vi "Reference_new version_1.0.vi"(1 "Phase log in":dbl=0.9999999999996251, 2 "AI Block Size":i32=40000, 4 "Phase&time":T1, 5 "Reset":bool, 6 "Frequency":dbl=20.0 format="%.2f", 7 "Ref Shape":enum16{"Sine", "Square"}(ring), 8 "Ref Amp":dbl=5.0 format="%.2f", 9 "AI Rate":dbl=200000.0) -> (0 "Ref out":T2={"Ref X"=array[40000 elements], "Ref Y"=array[40000 elements], "AI Rate"=200000.0, "AI Block Size"=40000.0, "Frequency"=20.0, "Ref amp"=5.0} {"Ref amp" step=0.001 format="%0.4f"; "Frequency" step=0.001 format="%0.4f"; "AI Block Size" step=0.001 format="%0.4f"; "AI Rate" step=0.001 format="%0.4f"}, 3 "Phase log":dbl=0.9999999999996251)   [LabVIEW 2013]
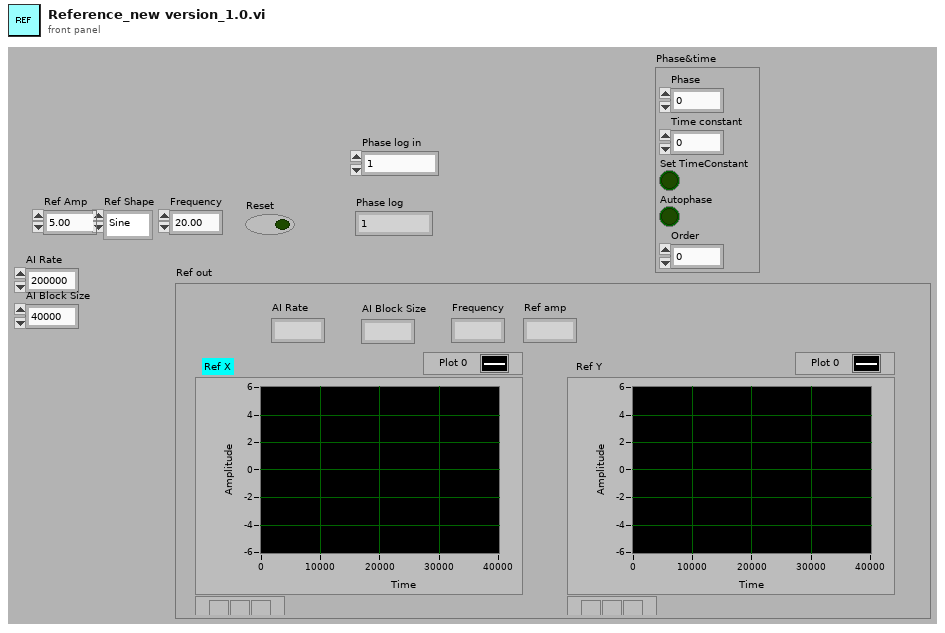
[diagram p1: front panel]
types:
  T1 = cluster{"Phase":dbl, "Time constant":dbl, "Set TimeConstant":bool, "Autophase":bool, "Order":dbl}
  T2 = cluster{"Ref X":dbl[], "Ref Y":dbl[], "AI Rate":dbl, "AI Block Size":dbl, "Frequency":dbl, "Ref amp":dbl}
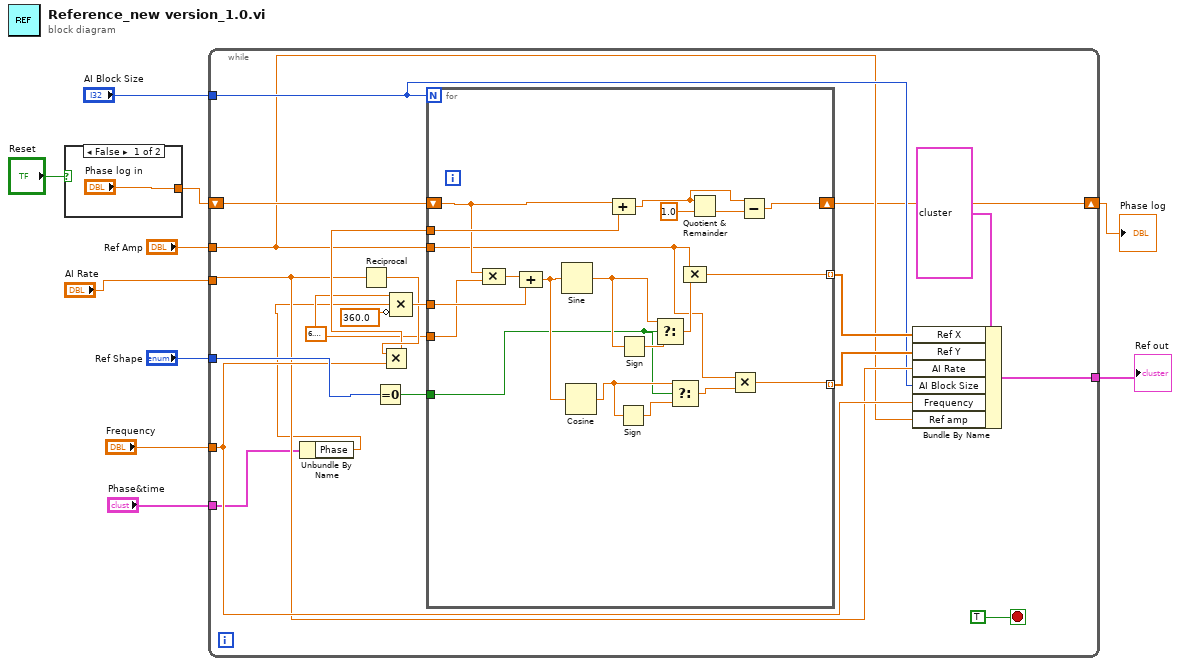
[diagram p0: block diagram]
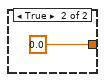
[diagram p2: hidden frame]
diagram:
  n1 = case shown="False" "Reset" {
    tunnel: ["Phase log in" 0.0] -> w7
    frame False {
    }
    frame True {
    }
  }
  n2 = while {
    shift-left: w7 -> [w32]
    shift-right: [w16] -> w5
    tunnel: "AI Block Size" -> [w19]
    tunnel: "Ref Amp" -> [w18]
    tunnel: "AI Rate" -> [w20]
    tunnel: "Ref Shape" -> [w27]
    tunnel: "Frequency" -> [w21]
    tunnel: "Phase&time" -> [w15]
    tunnel: [w13] -> w1
    stop <- TRUE stop-if-true
    w24 = 6.283185307179586
    n3 = Unbundle By Name(w15) -> ("Phase"=w17:dbl)
    n4 = Reciprocal(x=w20) -> (1/x=w26:dbl)
    n5 = Equal To 0?(x=w27) -> (x = 0?=w30:bool)
    n6 = Multiply(x=w26, y=w21) -> (x*y=w25:dbl)
    n7 = Compound Arithmetic op=MULTIPLY(w17, w24, invert 360.0 ("value")) -> (w29:dbl)
    n8 = for {
      N: w19 -> [_]
      shift-right: [w41] -> w16
      shift-left: w32 -> [w46]
      tunnel: w25 -> [w52]
      tunnel: w18 -> [w34]
      tunnel: w30 -> [w36]
      tunnel: w29 -> [w49]
      tunnel: [w45] -> w23 mode=indexing
      tunnel: w24 -> [w40]
      tunnel: [w33] -> w22 mode=indexing
      n9 = Compound Arithmetic op=MULTIPLY(w46, w40) -> (w50:dbl)
      n10 = Compound Arithmetic op=ADD(w50, w49) -> (w39:dbl)
      n11 = Sine(x=w39) -> (sin(x)=w48:dbl)
      n12 = Cosine(x=w39) -> (cos(x)=w38:dbl)
      n13 = Compound Arithmetic op=ADD(w46, w52) -> (w43:dbl)
      n14 = Sign(1:w38) -> (0:w37:dbl)
      n15 = Sign(1:w48) -> (0:w47:dbl)
      n16 = Select(t=w48, s=w36, f=w47) -> (s? t:f=w51:dbl)
      n17 = Select(t=w38, s=w36, f=w37) -> (s? t:f=w35:dbl)
      n18 = Compound Arithmetic op=MULTIPLY(w34, w51) -> (w45:dbl)
      n19 = Quotient & Remainder(x=w43, y=1.0) -> (floor(x/y)=w42:dbl)  [unwired: 1 out]
      n20 = Multiply(x=w34, y=w35) -> (x*y=w33:dbl)
      n21 = Subtract(x=w43, y=w42) -> (x-y=w41:dbl)
    }
    n22 = Bundle By Name(cluster=T2 {"Ref X"=array[40000 elements], "Ref Y"=array[40000 elements], "AI Rate"=200000.0, "AI Block Size"=40000.0, "Frequency"=20.0, "Ref amp"=5.0} ("Ref out"), "Ref X"=w23, "Ref Y"=w22, "AI Rate"=w20, "AI Block Size"=w19, "Frequency"=w21, "Ref amp"=w18) -> (w13:T2)
  }
  "Phase log" <- w5
  "Ref out" <- w1
